vi "water monitoring.vi"() -> ()   [LabVIEW 2022 SP3]
panel:
  out "Boolean 4":bool caption="Boolean"
  out "Boolean 3":bool caption="Boolean"
  out "Boolean 2":bool caption="Boolean"
  out "Boolean":bool
  out "String 4":string
  in  "TDS":dbl(knob) scale=0.0..1000.0
  out "Drain 2":bool
  out "String 3":string
  out "String 2":string
  in  "TURBIDITY SENSOR":dbl(slide) scale=0.0..15.0
  out "Drain":bool
  out "Caution":bool
  out "Safe":bool
  out "Drain":bool
  out "String":string
  out "Pump":bool
  in  "PH SENSOR":dbl(knob) min=0.0 max=14.0 step=1.0 scale=0.0..14.0
  in  "Tank":dbl(slide) scale=0.0..100.0
  in  "Float Switch":bool
  in  "stop":bool
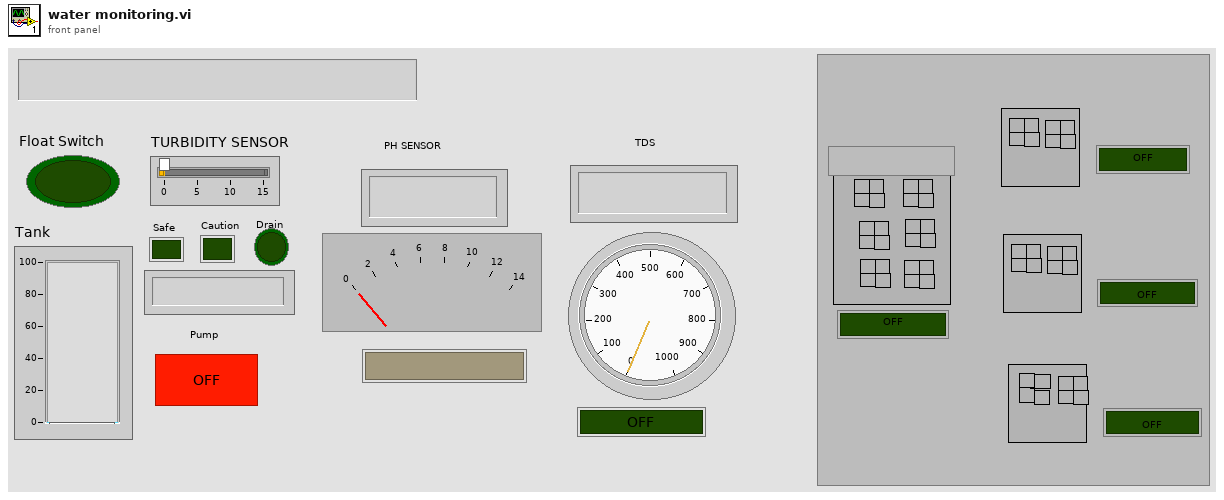
[diagram p1: front panel]
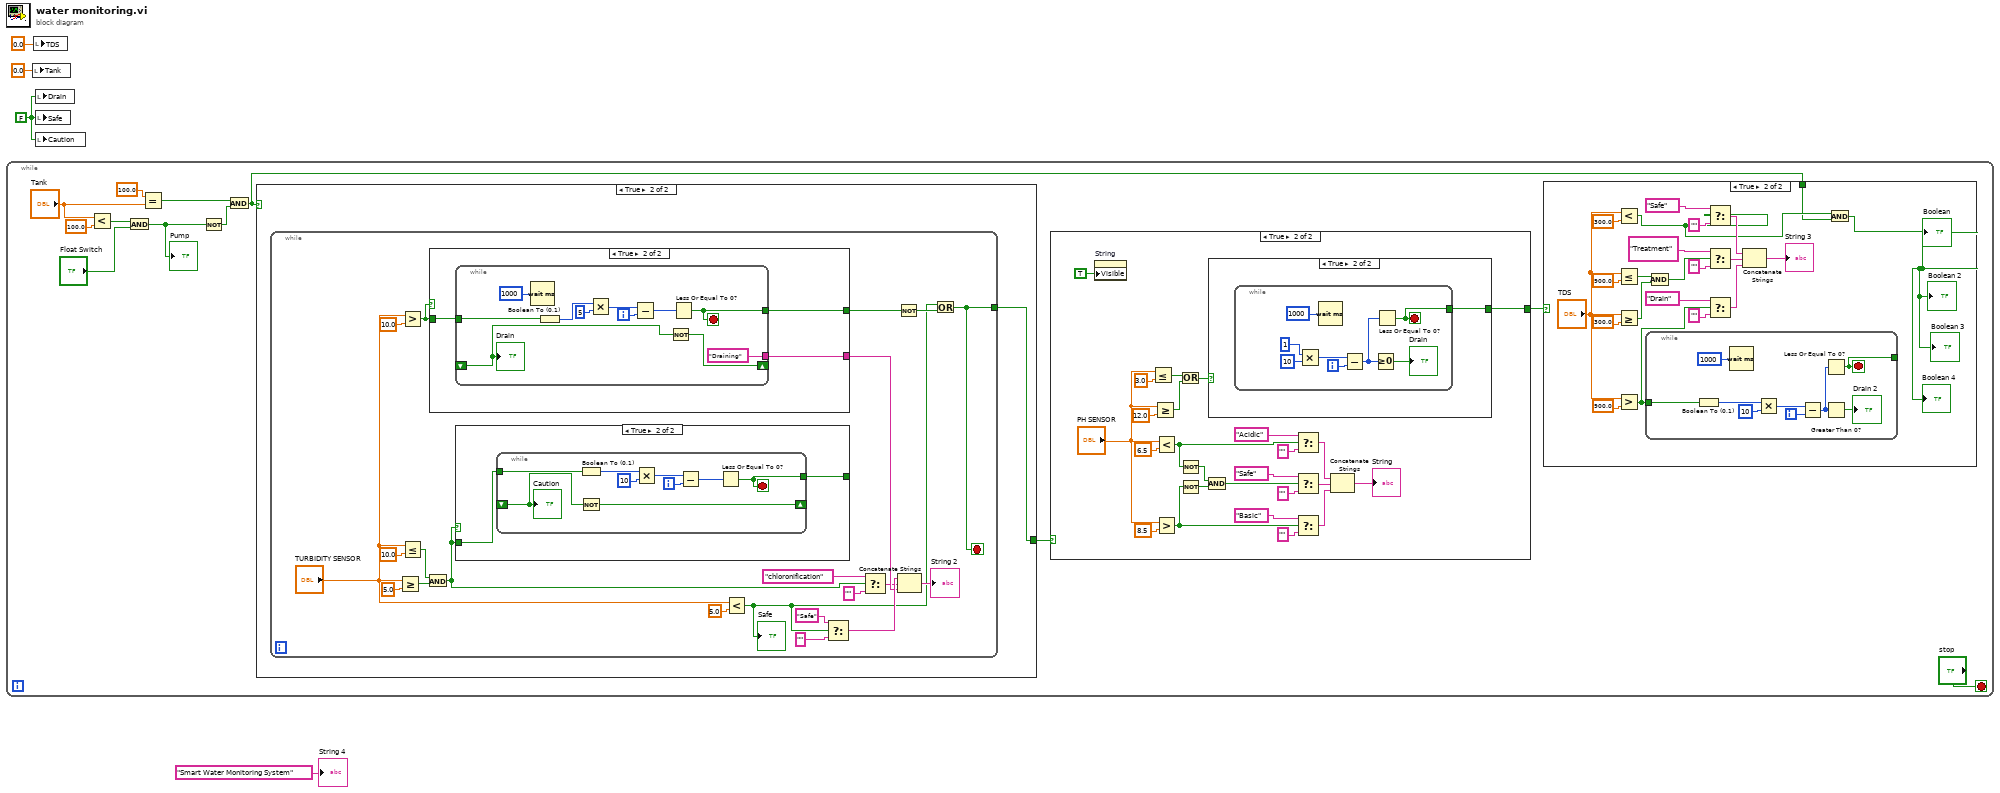
[diagram p0: block diagram]
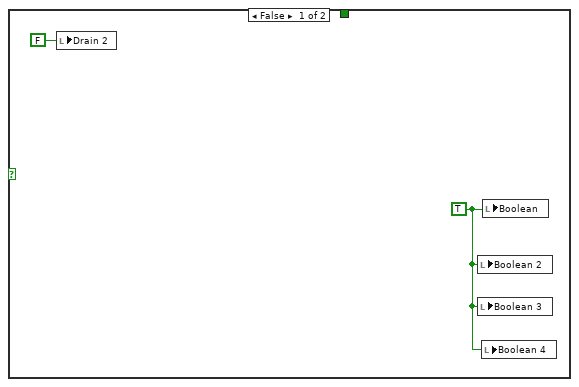
[diagram p2: hidden frame]
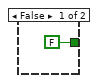
[diagram p3: hidden frame]
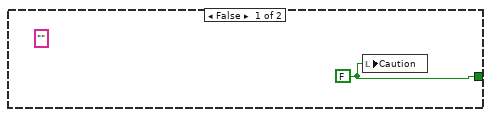
[diagram p4: hidden frame]
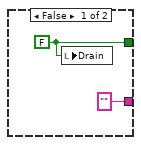
[diagram p5: hidden frame]
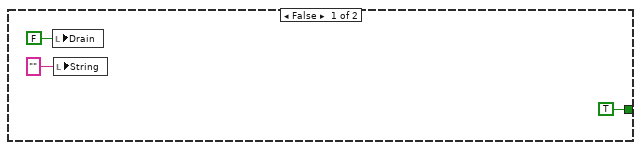
[diagram p6: hidden frame]
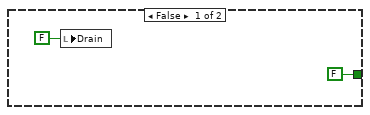
[diagram p7: hidden frame]
diagram:
  w3 = FALSE ("Safe")
  n1 = while {
    stop <- "stop" stop-if-true
    n2 = Less?(x="Tank", y=100.0) -> (x < y?=w15:bool)
    n3 = And(x=w15, y="Float Switch") -> (x .and. y?=w12:bool)
    "Pump" <- w12
    n4 = Equal?(x=100.0, y="Tank") -> (x = y?=w9:bool)
    n5 = Not(x=w12) -> (.not. x?=w8:bool)
    n6 = And(x=w9, y=w8) -> (x .and. y?=w5:bool)
    n7 = case shown="True" w5 {
      tunnel: [FALSE w51] -> w7
      frame False {
      }
      frame True {
        n8 = while {
          tunnel: [w53] -> w51
          stop <- w53 stop-if-true
          n9 = Greater Or Equal?(x="TURBIDITY SENSOR", y=5.0) -> (x >= y?=w69:bool)
          n10 = Greater?(x="TURBIDITY SENSOR", y=10.0) -> (0:w61:bool)
          n11 = Less Or Equal?(x="TURBIDITY SENSOR", y=10.0) -> (x <= y?=w68:bool)
          n12 = And(x=w68, y=w69) -> (x .and. y?=w57:bool)
          n13 = case shown="True" w61 {
            tunnel: w61 -> [_ w89]
            tunnel: ["" w88] -> w60
            tunnel: [w85 w87] -> w59
            frame False {
              w85 = FALSE
              n14 = local write "Drain"(w85) -> ()
            }
            frame True {
              n15 = while {
                shift-right: [w97] -> _
                shift-left: _ -> [w96]
                tunnel: w89 -> [w95]
                tunnel: ["Draining"] -> w88
                tunnel: [w91] -> w87
                i -> [w94]
                stop <- w91 stop-if-true
                n16 = Wait (ms)(milliseconds to wait=u32 1000) -> ()  [unwired: 1 out]
                n17 = Boolean To (0,1)(Boolean=w95) -> (0, 1=w100:i16)
                n18 = Multiply(x=w100, y=i16 5) -> (x*y=w99:i16)
                n19 = Subtract(x=w99, y=w94) -> (x-y=w98:i32)
                n20 = Not(x=w96) -> (.not. x?=w97:bool)
                n21 = Less Or Equal To 0?(x=w98) -> (x <= 0?=w91:bool)
                "Drain" <- w96
              }
            }
          }
          n22 = case shown="True" w57 {
            tunnel: [w73 w75] -> _
            tunnel: w57 -> [_ w74]
            frame False {
              (unwired) ""
              w73 = FALSE ("Caution")
              n23 = local write "Caution"(w73) -> ()
            }
            frame True {
              n24 = while {
                shift-right: [w84] -> _
                shift-left: _ -> [w80]
                tunnel: [w78] -> w75
                tunnel: w74 -> [w76]
                i -> [w79]
                stop <- w78 stop-if-true
                n25 = Boolean To (0,1)(Boolean=w76) -> (0, 1=w81:i16)
                n26 = Not(x=w80) -> (.not. x?=w84:bool)
                n27 = Multiply(x=w81, y=i16 10) -> (x*y=w82:i16)
                n28 = Subtract(x=w82, y=w79) -> (x-y=w83:i32)
                n29 = Less Or Equal To 0?(x=w83) -> (x <= 0?=w78:bool)
                "Caution" <- w80
              }
            }
          }
          n30 = Less?(x="TURBIDITY SENSOR", y=5.0) -> (x < y?=w52:bool)
          "Safe" <- w52
          n31 = Select(t="Safe", s=w52, f="") -> (s? t:f=w65:string)
          n32 = Select(t="chloronification", s=w57, f="") -> (s? t:f=w54:string)
          n33 = Not(x=w59) -> (.not. x?=w58:bool)
          n34 = Concatenate Strings(w65, w54, w60) -> (→"String 2":string)
          n35 = Or(x=w52, y=w58) -> (x .or. y?=w53:bool)
        }
      }
    }
    n36 = case shown="True" w7 {
      tunnel: [TRUE w105] -> w6
      frame False {
        n37 = local write "Drain"(FALSE) -> ()
        n38 = local write "String"("" ("String")) -> ()
      }
      frame True {
        n39 = property on="String" class="Str"("Visible"=TRUE) -> ()  [unwired: 2 in, 2 out]
        n40 = Less Or Equal?(x="PH SENSOR", y=3.0) -> (x <= y?=w110:bool)
        n41 = Greater Or Equal?(x="PH SENSOR", y=12.0) -> (x >= y?=w109:bool)
        n42 = Less?(x="PH SENSOR", y=6.5) -> (x < y?=w112:bool)
        n43 = Greater?(x="PH SENSOR", y=8.5) -> (0:w117:bool)
        n44 = Or(x=w110, y=w109) -> (x .or. y?=w108:bool)
        n45 = Not(x=w112) -> (.not. x?=w127:bool)
        n46 = Not(x=w117) -> (.not. x?=w128:bool)
        n47 = And(x=w127, y=w128) -> (x .and. y?=w120:bool)
        n48 = case shown="True" w108 {
          tunnel: [FALSE w131] -> w105
          frame False {
            n49 = local write "Drain"(FALSE ("Drain")) -> ()
          }
          frame True {
            n50 = while {
              tunnel: [w132] -> w131
              i -> [w137]
              stop <- w132 stop-if-true
              n51 = Multiply(x=i16 1 ("y"), y=i16 10) -> (x*y=w138:i16)
              n52 = Wait (ms)(milliseconds to wait=u32 1000) -> ()  [unwired: 1 out]
              n53 = Subtract(x=w138, y=w137) -> (x-y=w135:i32)
              n54 = Greater Or Equal To 0?(x=w135) -> (x >= 0?=→"Drain":bool)
              n55 = Less Or Equal To 0?(x=w135) -> (x <= 0?=w132:bool)
            }
          }
        }
        n56 = Select(t="Acidic", s=w112, f="") -> (s? t:f=w122:string)
        n57 = Select(t="Safe", s=w120, f="") -> (s? t:f=w113:string)
        n58 = Select(t="Basic", s=w117, f="") -> (s? t:f=w114:string)
        n59 = Concatenate Strings(w122, w113, w114) -> (→"String":string)
      }
    }
    n60 = case shown="True" w6 {
      tunnel: w5 -> [_ w19]
      frame False {
        w17 = TRUE
        n61 = local write "Drain 2"(FALSE ("Drain 2")) -> ()
        n62 = local write "Boolean 2"(w17) -> ()
        n63 = local write "Boolean 3"(w17) -> ()
        n64 = local write "Boolean 4"(w17) -> ()
        n65 = local write "Boolean"(w17) -> ()
      }
      frame True {
        n66 = Less?(x="TDS", y=300.0) -> (x < y?=w20:bool)
        n67 = Less Or Equal?(x="TDS", y=900.0) -> (x <= y?=w39:bool)
        n68 = Greater Or Equal?(x="TDS", y=300.0) -> (x >= y?=w40:bool)
        n69 = Greater?(x="TDS", y=900.0) -> (0:w23:bool)
        n70 = while {
          tunnel: [w43] -> _
          tunnel: w23 -> [w41]
          i -> [w47]
          stop <- w43 stop-if-true
          n71 = Boolean To (0,1)(Boolean=w41) -> (0, 1=w42:i16)
          n72 = Wait (ms)(milliseconds to wait=u32 1000) -> ()  [unwired: 1 out]
          n73 = Multiply(x=w42, y=i16 10) -> (x*y=w48:i16)
          n74 = Subtract(x=w48, y=w47) -> (x-y=w45:i32)
          n75 = Less Or Equal To 0?(x=w45) -> (x <= 0?=w43:bool)
          n76 = Greater Than 0?(x=w45) -> (x > 0?=→"Drain 2":bool)
        }
        n77 = And(x=w39, y=w40) -> (x .and. y?=w24:bool)
        n78 = Select(t="Safe", s=w20, f="") -> (s? t:f=w27:string)
        n79 = Select(t="Treatment", s=w24, f="") -> (s? t:f=w34:string)
        n80 = Select(t="Drain", s=w23, f="") -> (s? t:f=w33:string)
        n81 = Concatenate Strings(w27, w34, w33) -> (→"String 3":string)
        n82 = And(x=w20, y=w19) -> (x .and. y?=→"Boolean 2" →"Boolean 3" →"Boolean 4" →"Boolean":bool)
      }
    }
  }
  n83 = local write "Tank"(0.0 ("Tank 3")) -> ()
  n84 = local write "TDS"(0.0 ("Gauge")) -> ()
  n85 = local write "Drain"(w3) -> ()
  n86 = local write "Safe"(w3) -> ()
  n87 = local write "Caution"(w3) -> ()
  "String 4" <- "Smart Water Monitoring System" ("String 4")
